vi "find_mouse_coords.vi"(2 "XYGraph in":refnum<vi>, 3 "mouse coords":T1) -> (1 "coords in plot":cluster{"x value":dbl, "y value":dbl})   [LabVIEW 2017]
doc: "finds the coordinates of the mouse click inside a plot. the coordinates are give in plot-data-inuts and not in pixels. Can be used to set a cursor."
uses:
  <vilib>/Utility/miscctls.llb/LVPoint32TypeDef.ctl
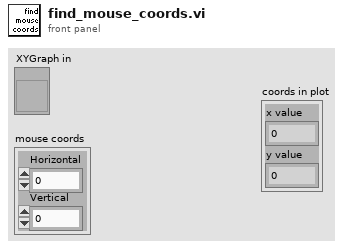
[diagram p1: front panel]
types:
  T1 = typedef "LVPoint32TypeDef.ctl" = cluster{"Horizontal":i32, "Vertical":i32}
  T2 = typedef "LVRectTypeDef.ctl" = cluster{"Left":i16, "Top":i16, "Right":i16, "Bottom":i16}
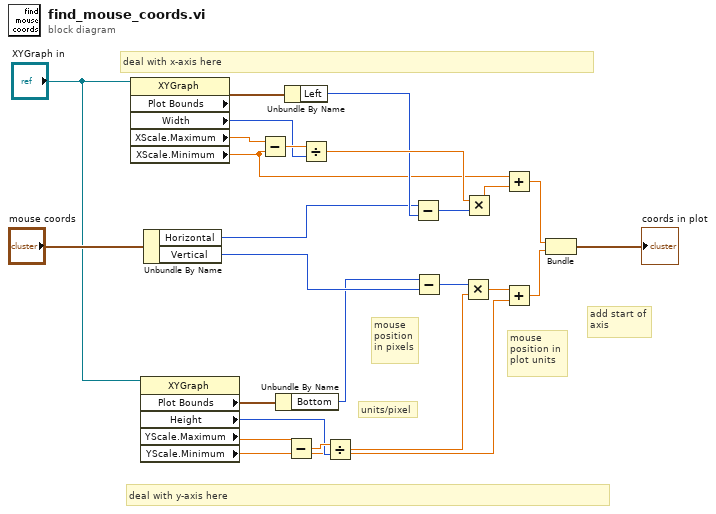
[diagram p0: block diagram]
diagram:
  # "deal with y-axis here"
  # "deal with x-axis here"
  # "add start of\naxis"
  # "mouse\nposition in\nplot units"
  # "mouse\nposition\nin pixels"
  # "units/pixel"
  n1 = property on="Property Node" class="XYGraph"(reference="XYGraph in") -> ("Plot Bounds"=w15:T2, "Width"=w3:u32, "XScale.Maximum"=w2:dbl, "XScale.Minimum"=w1:dbl)  [unwired: 1 in, 2 out]
  n2 = property on="Property Node" class="XYGraph"(reference="XYGraph in") -> ("Plot Bounds"=w11:T2, "Height"=w8:u32, "YScale.Maximum"=w10:dbl, "YScale.Minimum"=w5:dbl)  [unwired: 1 in, 2 out]
  n3 = Unbundle By Name("mouse coords") -> ("Horizontal"=w14:i32, "Vertical"=w25:i32)
  n4 = Subtract(x=w2, y=w1) -> (x-y=w19:dbl)
  n5 = Unbundle By Name(w11) -> ("Bottom"=w4:i16)
  n6 = Unbundle By Name(w15) -> ("Left"=w16:i16)
  n7 = Subtract(x=w10, y=w5) -> (x-y=w9:dbl)
  n8 = Divide(x=w19, y=w3) -> (x/y=w20:dbl)
  n9 = Divide(x=w9, y=w8) -> (x/y=w6:dbl)
  n10 = Subtract(x=w14, y=w16) -> (x-y=w18:i32)
  n11 = Subtract(x=w4, y=w25) -> (x-y=w7:i32)
  n12 = Multiply(x=w7, y=w6) -> (x*y=w23:dbl)
  n13 = Multiply(x=w20, y=w18) -> (x*y=w21:dbl)
  n14 = Add(x=w1, y=w21) -> (x+y=w22:dbl)
  n15 = Add(x=w23, y=w5) -> (x+y=w24:dbl)
  n16 = Bundle(w22, w24) -> (→"coords in plot":cluster{dbl, dbl})  [unwired: 1 in]
